vi "Read.vi"(8 "error in (no error)":errorcluster, 11 "CryoCoolerAVC in":refnum<class "CryoCoolerAVC.lvclass">) -> (0 "error out":errorcluster, 2 "Data":dbl[](array[numeric]), 3 "CryoCoolerAVC out":refnum<class "CryoCoolerAVC.lvclass">)   [LabVIEW 2024, in "CryoCoolerAVC.lvclass"]
uses:
  CryoCoolerAVC.lvclass
  CryoCoolerAVC.lvclass/CryoCoolerAVC.ctl
  Cryo Cooler.lvclass
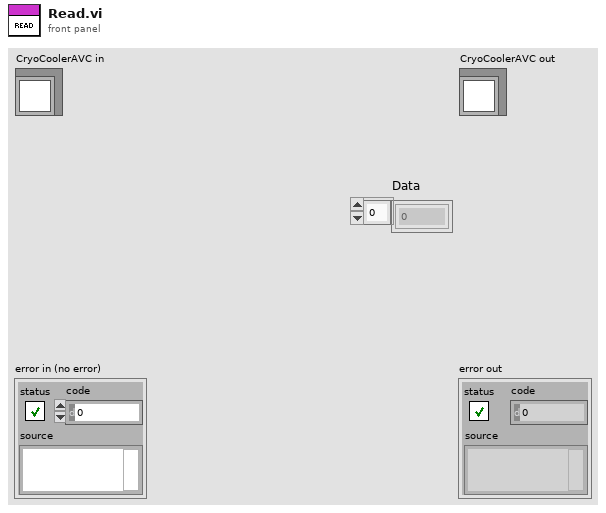
[diagram p1: front panel]
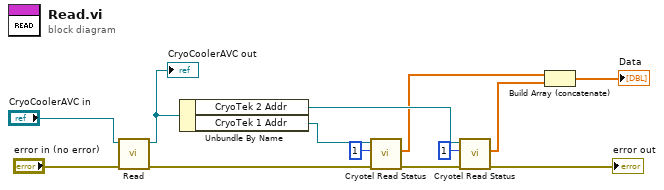
[diagram p0: block diagram]
diagram:
  n1 = call-parent "Read.vi"("error in (no error)"="error in (no error)", "Cryo Cooler in"="CryoCoolerAVC in") -> ("error out"=w11:errorcluster, "Cryo Cooler out"=w10:refnum<class "CryoCoolerAVC.lvclass">)  [unwired: 7 in, 1 out]
  "CryoCoolerAVC out" <- w10
  n2 = Unbundle By Name(w10) -> ("CryoTek 2 Addr"=w7:refnum<visa-resource-name>, "CryoTek 1 Addr"=w9:refnum<visa-resource-name>)
  n3 = call "Cryotel Read Status.vi"("error in"=w11, "Number of reads"=1, "VISA Resource (write)"=w9) -> ("error out"=w5:errorcluster, "Data"=w4:dbl[])  [unwired: 6 in, 1 out]
  n4 = call "Cryotel Read Status.vi"("error in"=w5, "Number of reads"=1, "VISA Resource (write)"=w7) -> ("error out"=→"error out":errorcluster, "Data"=w3:dbl[])  [unwired: 6 in, 1 out]
  n5 = Build Array (concatenate)(w4, w3) -> (→"Data":dbl[])
